vi "Text to StringArray.vi"(1 "String":string) -> (0 "array":string[](array[string]))   [LabVIEW 2020]
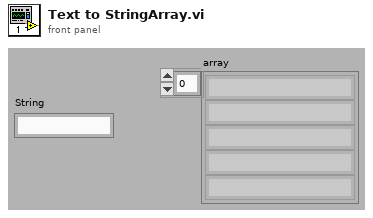
[diagram p1: front panel]
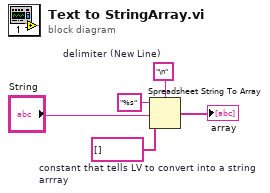
[diagram p0: block diagram]
diagram:
  w2 = "\n"  # delimiter (New Line)
  w5 = string[] []  # constant that tells LV to convert into a string arrray
  n1 = Spreadsheet String To Array(delimiter (Tab)=w2, format string="%s", spreadsheet string="String", array type (2D Dbl)=w5) -> (array=→"array":string[])
